vi "open.vi"(8 "error in (no error)":errorcluster, 11 "SoundAO in":refnum<class "SoundAO.lvclass">) -> (0 "error out":errorcluster, 3 "SoundAO out":refnum<class "SoundAO.lvclass">)   [LabVIEW 2009, in "Hardware.lvlib" / "Channels.lvlib" / "SoundAO.lvclass"]
uses:
  SoundAO.lvclass
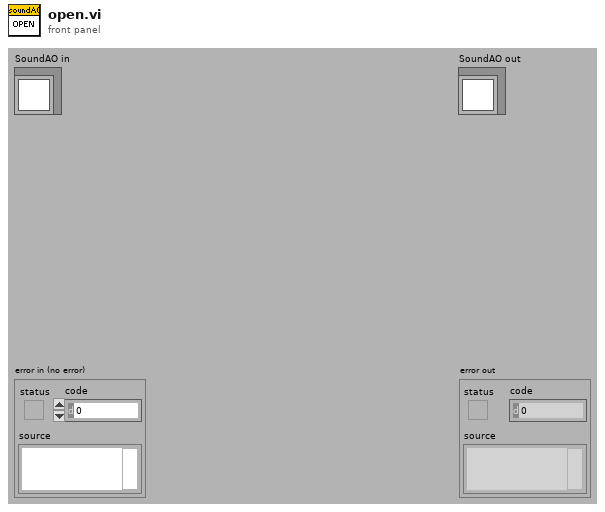
[diagram p1: front panel]
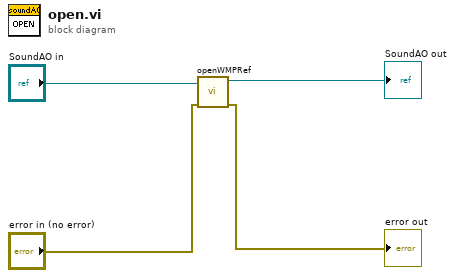
[diagram p0: block diagram]
diagram:
  n1 = call "openWMPRef.vi"("error in (no error)"="error in (no error)", "SoundAO in"="SoundAO in") -> ("error out"=→"error out":errorcluster, "SoundAO out"=→"SoundAO out":refnum<class "SoundAO.lvclass">)  [unwired: 8 in]
